vi "SPD.PowerSource Test.vi"(8 "Error In":errorcluster, 11 "SPD.Stand Ctrl in":T1 {"spdDeviceSession"."hidSPD.Sturtup Values"."HV_bias" format="%#_6p, V"; "spdDeviceSession"."hidSPD.Sturtup Values"."TSet" format="%#_6p, DegC"; "spdDeviceSession"."hidSPD.Controller"."HV_bias" format="%#_6p, V"; "spdDeviceSession"."hidSPD.Controller"."TSet" format="%#_6p, DegC"}) -> (0 "Error Out":errorcluster, 1 "ok":bool, 3 "SPD.Stand Ctrl out":T1 {"spdDeviceSession"."hidSPD.Sturtup Values"."HV_bias" format="%#_6p, V"; "spdDeviceSession"."hidSPD.Sturtup Values"."TSet" format="%#_6p, DegC"; "spdDeviceSession"."hidSPD.Controller"."HV_bias" format="%#_6p, V"; "spdDeviceSession"."hidSPD.Controller"."TSet" format="%#_6p, DegC"})   [LabVIEW 2018]
uses:
  typedefs/SPD.Stand Ctrl.ctl
  Instruments/SPD HID Interface/hidSPDLibForLabView/LibVIs/hidSPD Controls/hidSPD Device Session.ctl
  Instruments/SPD HID Interface/hidSPDLibForLabView/LibVIs/hidSPD Controls/hidSPD Controller.ctl
  Instruments/SPD HID Interface/hidSPDLibForLabView/LibVIs/hidSPD Controls/hidSPD SPD Type.ctl
  Instruments/KC705 DevBoard/typedefs/DevB.Session.ctl
  Instruments/KeySight 53230A/typedefs/FreqC.Session.ctl
  Instruments/KeySight 8164B/KeySight 8164B LAN InstrLib/typedefs/KeySight 8164B control.ctl
  Instruments/LeCroy SDA830/typedefs/LeCroy.Session.ctl
  typedefs/SPD.Events.ctl
  ConfigFile/SPD.Config File ctrl.ctl
  <vilib>/Utility/config.llb/Config Data RefNum.ctl
  typedefs/SPD.Meas Result.ctl
  typedefs/SPD.Queues.ctl
  typedefs/SPD.Stand state.ctl
  Instruments/KeySight 8164B/KeySight 8164B LAN InstrLib.lvlib
  <vilib>/Utility/config.llb/NI_LVConfig.lvlib
  Instruments/SPD HID Interface/hidSPDLibForLabView/hidSPDLibForLabView.lvlib
panel:
  in  "Yes":bool
  in  "No":bool
  # "Источник питания подклячен в соответствии \nсо схемой подключения?\nНапряжение и ток выставлены правильно?"
  # "Схема подключения должна быть тут"
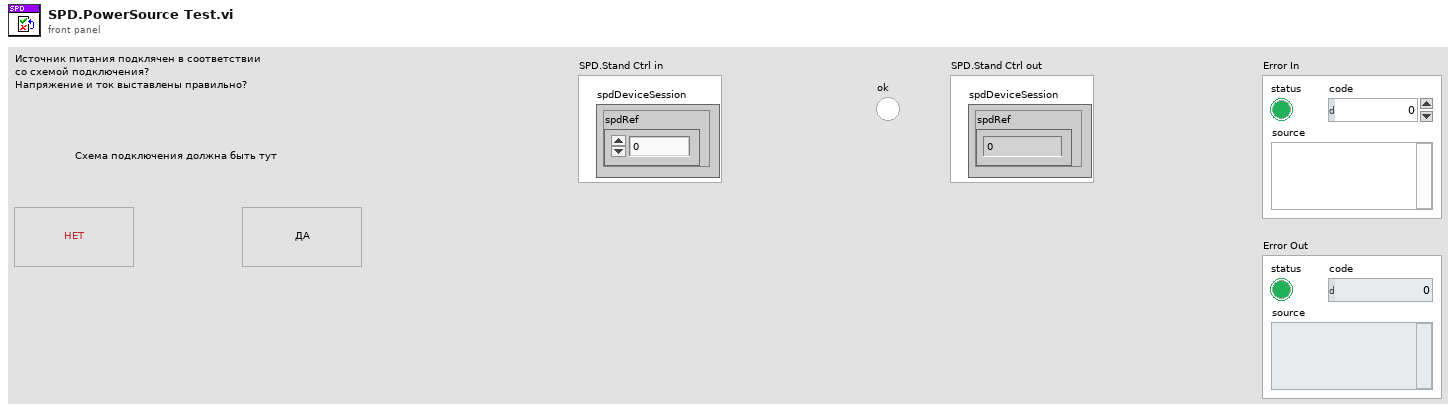
[diagram p1: front panel]
types:
  T1 = typedef "SPD.Stand Ctrl.ctl" = cluster{"spdDeviceSession":T2, "DevBSession":T5, "FreqCSession":T6, "8164BSession":T7, "LeCroySession":T8, "Events":T9, "configFile":T10, "SPD.Result":T12, "SPD.Queues":T13, "Console":refnum<vi>}
  T2 = typedef "hidSPDLibForLabView.lvlib/hidSPD Device Session.ctl" = cluster{"spdRef":u64, "connected":bool, "spdName":string, "hidSPD.Controller":T3, "hidSPD.Sturtup Values":T3, "SPD Type":T4}
  T3 = typedef "hidSPDLibForLabView.lvlib/hidSPD Controller.ctl" = cluster{"TSet":sgl, "HV_bias":sgl, "DDS_stb_code":u16}
  T4 = typedef "hidSPDLibForLabView.lvlib/hidSPD SPD Type.ctl" = enum16{"Free Run", "Gate"}
  T5 = typedef "DevB.Session.ctl" = cluster{"DevBRef":refnum<visa-resource-name>, "connected":bool}
  T6 = typedef "FreqC.Session.ctl" = cluster{"FreqCRef":refnum<visa-resource-name>, "timeout":dbl, "Gate":dbl, "connected":bool}
  T7 = typedef "KeySight 8164B LAN InstrLib.lvlib/KeySight 8164B control.ctl" = cluster{"Connection ID":refnum<k5>, "Connected":bool, "Info":string, "Slots Info":string[]}
  T8 = typedef "LeCroy.Session.ctl" = cluster{"LeCroySession":refnum<visa-resource-name>, "connected":bool}
  T9 = typedef "SPD.Events.ctl" = cluster{"DCRTest":refnum<user-event>, "Stop":refnum<user-event>}
  T10 = typedef "SPD.Config File ctrl.ctl" = cluster{"configFile ref":T11, "configFile path":path, "equipmentFile ref":T11}
  T11 = typedef "NI_LVConfig.lvlib/Config Data RefNum.ctl" = refnum<k1>
  T12 = typedef "SPD.Meas Result.ctl" = cluster{"HV_Bias":dbl[][][], "Stb_code":dbl[], "Temprature":dbl[], "Data":dbl[][][][], "DateTime":string}
  T13 = typedef "SPD.Queues.ctl" = cluster{"state queue":refnum<queue>}
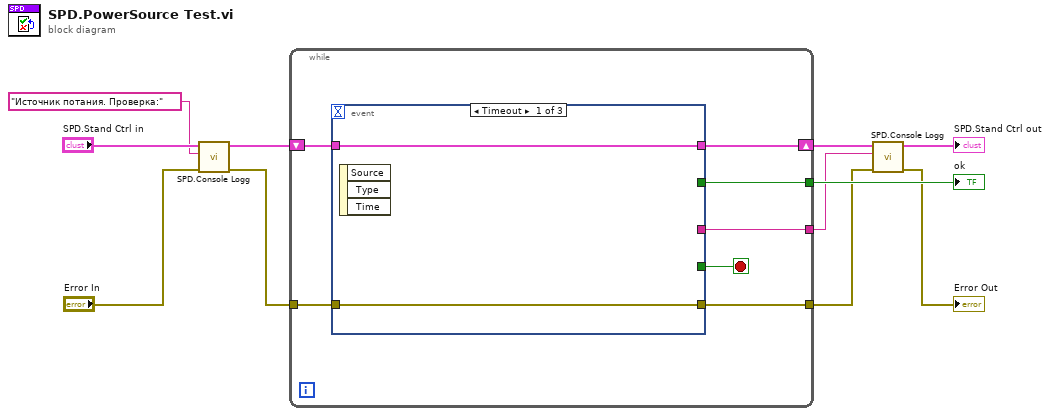
[diagram p0: block diagram]
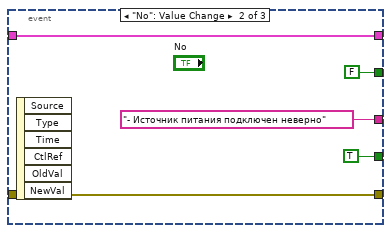
[diagram p2: hidden frame]
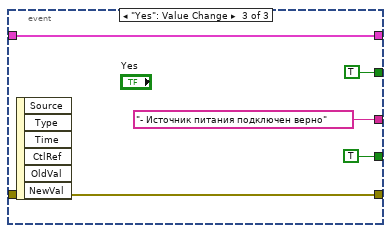
[diagram p3: hidden frame]
diagram:
  n1 = call "SPD.Console Logg.vi"("Error In"="Error In", "console Log"="Источник потания. Проверка:", "SPD.Stand Ctrl in"="SPD.Stand Ctrl in") -> ("Error Out"=w7:errorcluster, "SPD.Stand Ctrl out"=w9:T1)  [unwired: 7 in]
  n2 = while {
    shift-right: [w17] -> w5
    shift-left: w9 -> [w18]
    tunnel: w7 -> [w16]
    tunnel: [w15] -> w3
    tunnel: [w13] -> w11
    tunnel: [w12] -> w1
    stop <- w14 stop-if-true
    n3 = event shown="[0] Timeout" {
      selector: _ -> [_ _ _]
      dyn-events: _ -> [_ _ _]
      timeout: _ -> [_ _ _]
      tunnel: w18 -> [w20 w25 w30]
      tunnel: [w20 w25 w30] -> w17
      tunnel: [w19 w24 w29] -> w15
      tunnel: w16 -> [w19 w24 w29]
      tunnel: [_ TRUE TRUE] -> w14
      tunnel: [_ FALSE TRUE] -> w13
      tunnel: [_ "- Источник питания подключен неверно" ("report") "- Источник питания подключен верно" ("report")] -> w12
      event Timeout {
        n4 = event-data() -> ()  [unwired: 1 in, 3 out]
      }
      event "No": Value Change {
        n5 = event-data() -> ()  [unwired: 1 in, 6 out]
      }
      event "Yes": Value Change {
        n6 = event-data() -> ()  [unwired: 1 in, 6 out]
      }
    }
  }
  "ok" <- w11
  n7 = call "SPD.Console Logg.vi"("Error In"=w3, "console Log"=w1, "SPD.Stand Ctrl in"=w5) -> ("Error Out"=→"Error Out":errorcluster, "SPD.Stand Ctrl out"=→"SPD.Stand Ctrl out":T1)  [unwired: 7 in]
